vi "kjngeran.vi"() -> ()   [LabVIEW 2014]
panel:
  out "Grafic temperaturi":T1(graph)
  out "Temperatura curenta":u16
  out "Valoare convertita [V]":u16
  in  "Limita superioara":dbl
  in  "Limita inferioara":dbl
  in  "stop 2":bool
  out "comanda incalzitor":bool
  out "Temperatura medie":dbl(slide) scale=0.0..100.0
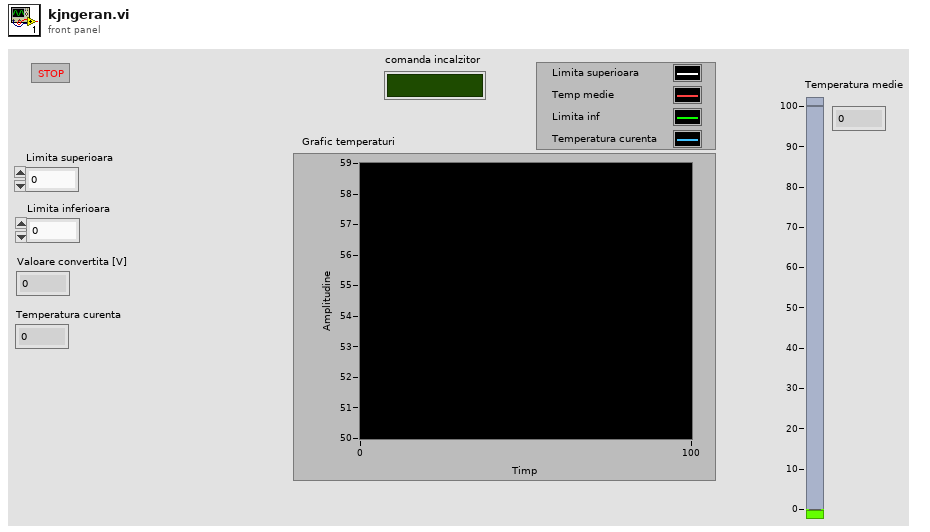
[diagram p1: front panel]
types:
  T1 = cluster{"Limita superioara":dbl, "Numeric":dbl, "Limita inferioara":dbl, dbl}
  T2 = cluster{"Limita superioara":dbl, dbl, "Limita inferioara":dbl, dbl}
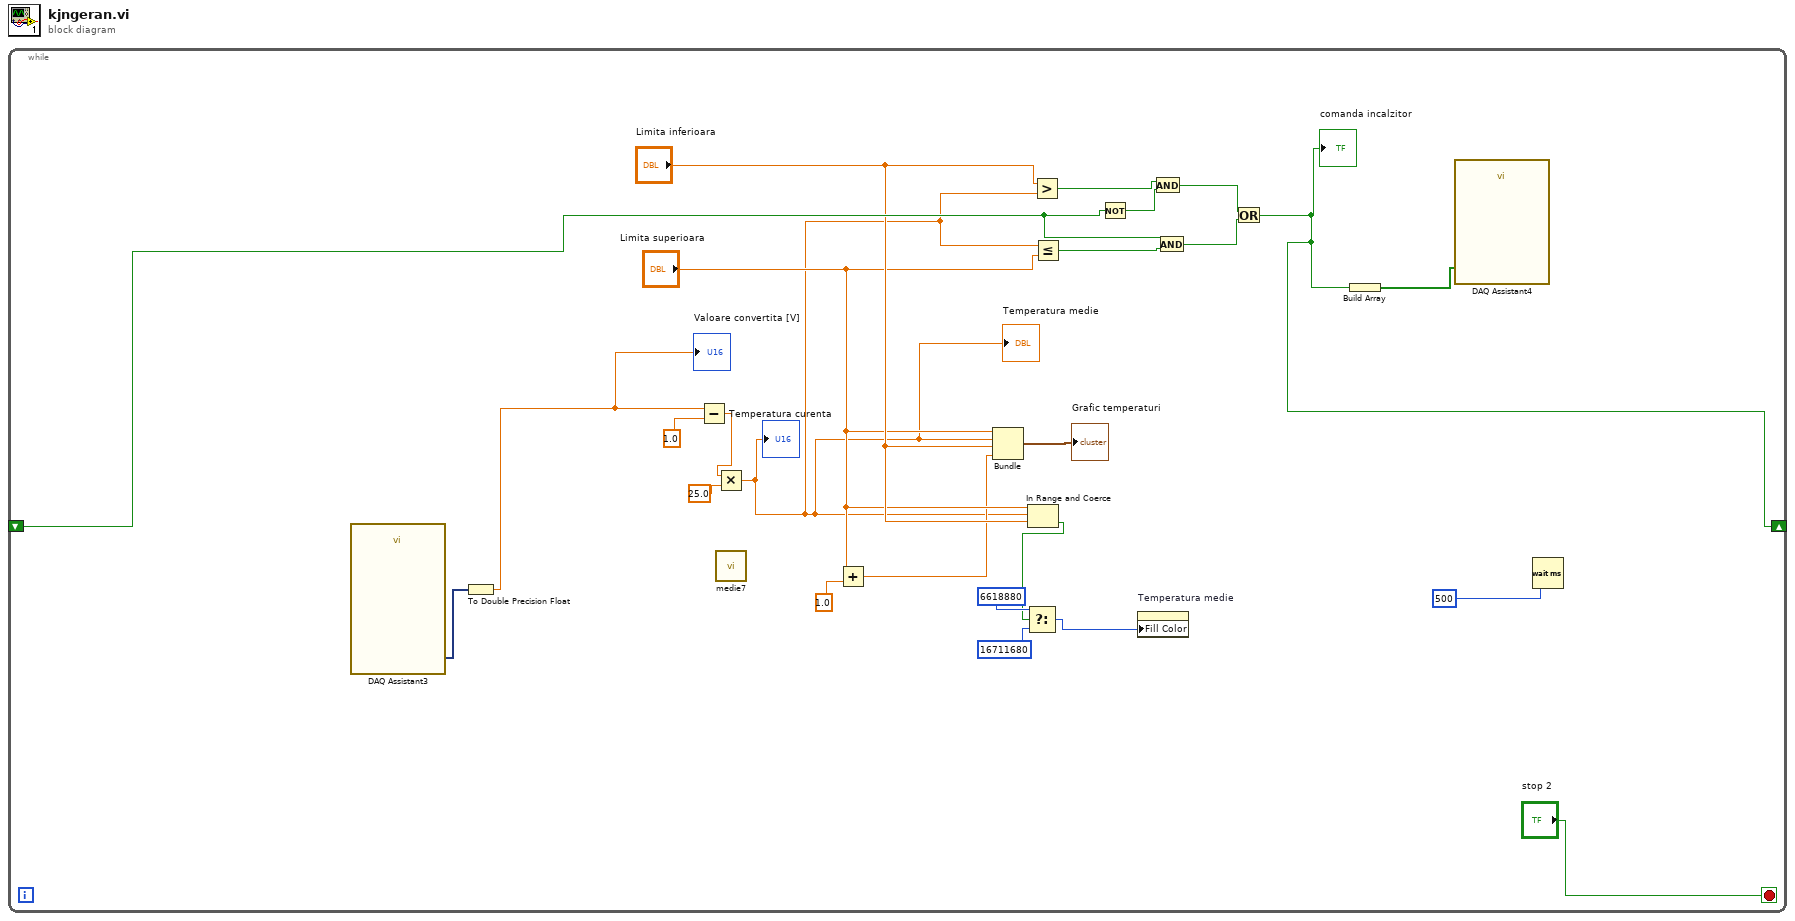
[diagram p0: block diagram]
diagram:
  n1 = while {
    shift-right: [w13] -> _
    shift-left: _ -> [w14]
    stop <- "stop 2" stop-if-true
    n2 = call "DAQ Assistant3"() -> ("data"=w24:dynamicdata)  [unwired: 17 in, 2 out]
    n3 = To Double Precision Float(number=w24) -> (double precision float=w3:dbl)
    "Valoare convertita [V]" <- w3
    n4 = Subtract(x=w3, y=1.0) -> (x-y=w21:dbl)
    n5 = Multiply(x=w21, y=25.0) -> (x*y=w1:dbl)
    "Temperatura curenta" <- w1
    "Temperatura medie" <- w1
    n6 = call "medie7.vi"() -> ()  [unwired: 11 in, 1 out]
    n7 = Add(x="Limita superioara", y=1.0) -> (x+y=w4:dbl)
    n8 = Bundle("Limita superioara"="Limita superioara", w1, "Limita inferioara"="Limita inferioara", w4) -> (→"Grafic temperaturi":T2)  [unwired: 1 in]
    n9 = In Range and Coerce(upper limit="Limita superioara", x=w1, lower limit="Limita inferioara") -> (In Range?=w9:bool)  [unwired: 1 out]
    n10 = Select(t=6618880, s=w9, f=16711680) -> (s? t:f=w2:i32)
    n11 = Greater?(x="Limita inferioara", y=w1) -> (0:w20:bool)
    n12 = Less Or Equal?(x=w1, y="Limita superioara") -> (x <= y?=w17:bool)
    n13 = Not(x=w14) -> (.not. x?=w15:bool)
    n14 = property on="Temperatura medie" class="Slide (strict)"("Fill Color"=w2) -> ()  [unwired: 2 in, 2 out]
    n15 = And(x=w20, y=w15) -> (x .and. y?=w19:bool)
    n16 = And(x=w14, y=w17) -> (x .and. y?=w16:bool)
    n17 = Or(x=w19, y=w16) -> (x .or. y?=w13:bool)
    "comanda incalzitor" <- w13
    n18 = Build Array(w13) -> (w18:bool[])
    n19 = call "DAQ Assistant4"("data"=w18) -> ()  [unwired: 17 in, 2 out]
    n20 = Wait (ms)(milliseconds to wait=500) -> ()  [unwired: 1 out]
  }
